vi "CreateTask.vi"(8 "error in (no error)":errorcluster, 9 "Tasks in":T5(c390), 10 "Cluster":cluster{"TaskName":string, "TaskConfig":T1} {"TaskConfig"."SampleRateConfiguration"."SampleMode" items=["Finite Samples"=10178, "Continuous Samples"=10123, "Hardware Timed Single Point"=12522]}, 11 "DAQ_Module in":refnum<class "DAQ_Module.lvclass">) -> (0 "error out":errorcluster, 1 "Tasks out":T5(c390), 3 "DAQ_Module out":refnum<class "DAQ_Module.lvclass">)   [LabVIEW 2025, in "DAQ_Module.lvlib" / "DAQ_Module.lvclass"]
uses:
  DAQ_Module.lvclass
  <vilib>/ActorFramework/Message Enqueuer/Message Enqueuer.lvclass
  DAQ_Task_Config.ctl
  DAQ_HW_Type.ctl
  DAQ_Task_Type.ctl
  DAQ_SampleRateConfig.ctl
  DAQ_Drive/NI_DAQmx/NI_DAQmx(AI)/NI_DAQmx(AI).lvclass
  DAQ_Module.lvclass/DAQ_Module.ctl
  D:/Hardware/DAQ/DAQ_Abstr/Task_Type/AI_Task/AI_Task/AI_Task.lvclass
  D:/Hardware/DAQ/DAQ_Abstr/Task_Abstr/Task_Abstr/Task_Abstr.lvclass
  C:/Program Files (x86)/National Instruments/LabVIEW 2025/vi.lib/ActorFramework/Actor/Actor.lvclass
  D:/Hardware/DAQ/DAQ_Drive/NI_DAQmx/NI_DAQmx(AI)/NI_DAQmx(AI).lvclass
  DAQ_Drive/NI_DAQmx/NI_DAQmx(Linear)/NI_DAQmx(Linear).lvclass
  D:/Hardware/DAQ/DAQ_Abstr/Task_Type/Linear_Task/Linear_Task/Linear_Task.lvclass
  D:/Hardware/DAQ/DAQ_Drive/NI_DAQmx/NI_DAQmx(Linear)/NI_DAQmx(Linear).lvclass
  DAQ_Abstr/Task_Abstr/Task_Abstr/Task_Abstr.lvclass
  D:/Hardware/DAQ/DAQ_Module/DAQ_Module/DAQ_Module/DAQ_Module.lvclass
  <vilib>/ActorFramework/Actor/Actor.lvclass
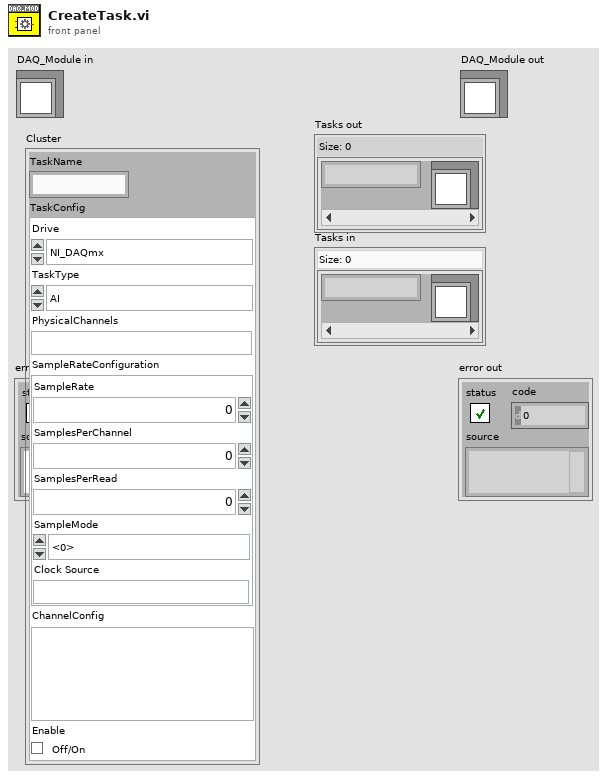
[diagram p1: front panel]
types:
  T1 = typedef "DAQ_Module.lvlib/DAQ_Module.lvclass/DAQ_Task_Config.ctl" = cluster{"Drive":T2, "TaskType":T3, "PhysicalChannels":string, "SampleRateConfiguration":T4, "ChannelConfig":string, "Enable":bool}
  T2 = typedef "DAQ_Module.lvlib/DAQ_Module.lvclass/DAQ_HW_Type.ctl" = enum16{"NI_DAQmx", "Simulated_DAQ"}
  T3 = typedef "DAQ_Module.lvlib/DAQ_Module.lvclass/DAQ_Task_Type.ctl" = enum16{"AI", "Linear", "Angular", "AO"}
  T4 = typedef "DAQ_Module.lvlib/DAQ_Module.lvclass/DAQ_SampleRateConfig.ctl" = cluster{"SampleRate":dbl, "SamplesPerChannel":u32, "SamplesPerRead":i32, "SampleMode":i32, "Clock Source":string}
  T5 = map{string, refnum<class "Message Enqueuer.lvclass">}
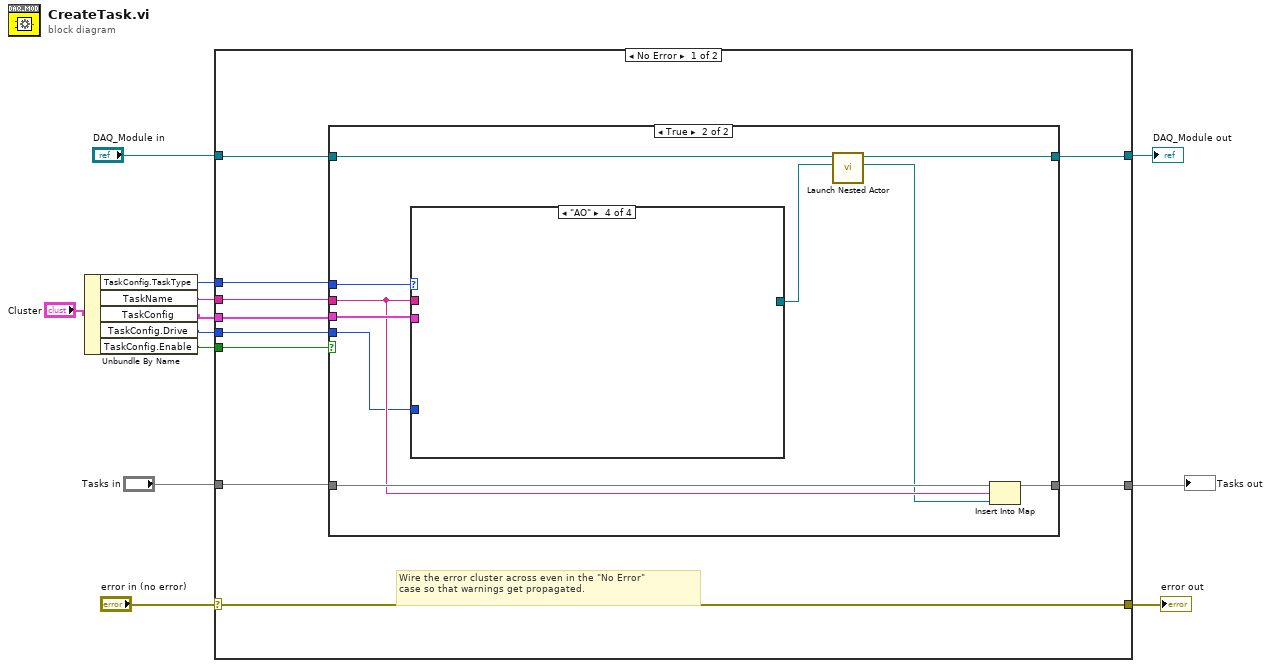
[diagram p0: block diagram]
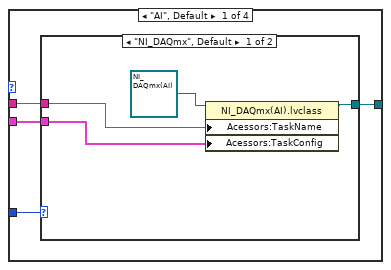
[diagram p3: hidden frame]
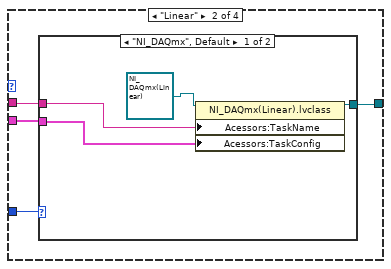
[diagram p5: hidden frame]
diagram:
  n1 = Unbundle By Name("Cluster") -> ("TaskConfig.TaskType"=w5:T3, "TaskName"=w4:string, "TaskConfig"=w3:T1, "TaskConfig.Drive"=w2:T2, "TaskConfig.Enable"=w1:bool)
  n2 = case shown="No Error" "error in (no error)" {
    selector: "error in (no error)" -> [w22 w53]
    tunnel: [w22 w53] -> w11
    tunnel: [w20 w52] -> w9
    tunnel: "DAQ_Module in" -> [w21 w52]
    tunnel: [w19 w51] -> w8
    tunnel: "Tasks in" -> [w18 w51]
    tunnel: w5 -> [w17 _]
    tunnel: w4 -> [w16 _]
    tunnel: w3 -> [w15 _]
    tunnel: w2 -> [w14 _]
    tunnel: w1 -> [w13 _]
    frame No Error {
      # "Wire the error cluster across even in the \"No Error\"\ncase so that warnings get propagated."
      n3 = case shown="True" w13 {
        tunnel: w21 -> [w24 w34]
        tunnel: [w24 w33] -> w20
        tunnel: w17 -> [_ w32]
        tunnel: w15 -> [_ w30]
        tunnel: w18 -> [w23 w29]
        tunnel: [w23 w28] -> w19
        tunnel: w16 -> [_ w27]
        tunnel: w14 -> [_ w25]
        frame False {
        }
        frame True {
          n4 = case shown="\"AO\"" w32 {
            tunnel: [w38 w43 _ _] -> w31
            tunnel: w27 -> [w37 w45 _ _]
            tunnel: w30 -> [w36 w44 _ _]
            tunnel: w25 -> [w35 w46 _ _]
            frame "AI", Default {
              n5 = case shown="\"NI_DAQmx\", Default" w35 {
                tunnel: [w41 _] -> w38
                tunnel: w37 -> [w40 _]
                tunnel: w36 -> [w39 _]
                frame "NI_DAQmx", Default {
                  n6 = property class="NI_DAQmx(AI).lvclass"(reference=refnum<class "NI_DAQmx(AI).lvclass"> refnum ("NI_DAQmx(AI).lvclass"), "Acessors:TaskName"=w40, "Acessors:TaskConfig"=w39) -> (reference out=w41:refnum<class "NI_DAQmx(AI).lvclass">)  [unwired: 1 in, 1 out]
                }
                frame "Simulated_DAQ" {
                }
              }
            }
            frame "Linear" {
              n7 = case shown="\"NI_DAQmx\", Default" w46 {
                tunnel: [w50 _] -> w43
                tunnel: w45 -> [w49 _]
                tunnel: w44 -> [w48 _]
                frame "NI_DAQmx", Default {
                  n8 = property class="NI_DAQmx(Linear).lvclass"(reference=refnum<class "NI_DAQmx(Linear).lvclass"> refnum ("NI_DAQmx(Linear).lvclass"), "Acessors:TaskName"=w49, "Acessors:TaskConfig"=w48) -> (reference out=w50:refnum<class "NI_DAQmx(Linear).lvclass">)  [unwired: 1 in, 1 out]
                }
                frame "Simulated_DAQ" {
                }
              }
            }
            frame "Angular" {
            }
            frame "AO" {
            }
          }
          n9 = call <vilib>:"Launch Nested Actor.vi"("Nested Actor"=w31, "Caller Actor in"=w34) -> ("Nested Actor's Enqueuer"=w26:refnum<class "Message Enqueuer.lvclass">, "Caller Actor in"=w33:refnum<class "DAQ_Module.lvclass">)  [unwired: 7 in, 1 out]
          n10 = Insert Into Map(map in=w29, key=w27, value=w26) -> (map out=w28:T5)  [unwired: 2 out]
        }
      }
    }
    frame Error {
    }
  }
  "error out" <- w11
  "DAQ_Module out" <- w9
  "Tasks out" <- w8
